vi "TCSLINK_global.vi"() -> ()   [LabVIEW 2015]
panel:
  out "Comp Mirror":bool
  in  "Dome":bool caption="Fe"
  out "Dome Percent":i8
  out "Quartz Percent":i8
  in  "Bulb":bool
  in  "Fe":bool
  in  "Quartz":bool
  in  "Ar":bool
  in  "Ne":bool
  in  "Cu":bool
  in  "Hg(Ar)":bool
  in  "Postion ADC":string
  in  "ObsDEC":string
  in  "ObsRA":string
  in  "Position Angle":dbl
  in  "Seeing":dbl
  in  "Humidity":dbl
  in  "Pressure":dbl
  in  "Wind Speed":dbl
  in  "Wind Direction":dbl
  in  "Outside Temp":dbl
  in  "Airmass":dbl
  in  "Focus":dbl
  in  "Rotator Location":string
  in  "Dome Shutter":string
  in  "Dome Az":dbl
  in  "Hour Angle":string
  in  "Sidereal Time":string
  in  "DEC":string
  in  "RA":string
  in  "Mount El":dbl
  in  "Mount Az":dbl
  in  "UT Time":string
  in  "Date":string
  in  "Rotator Angle":dbl
  out "TCSLink Online":bool
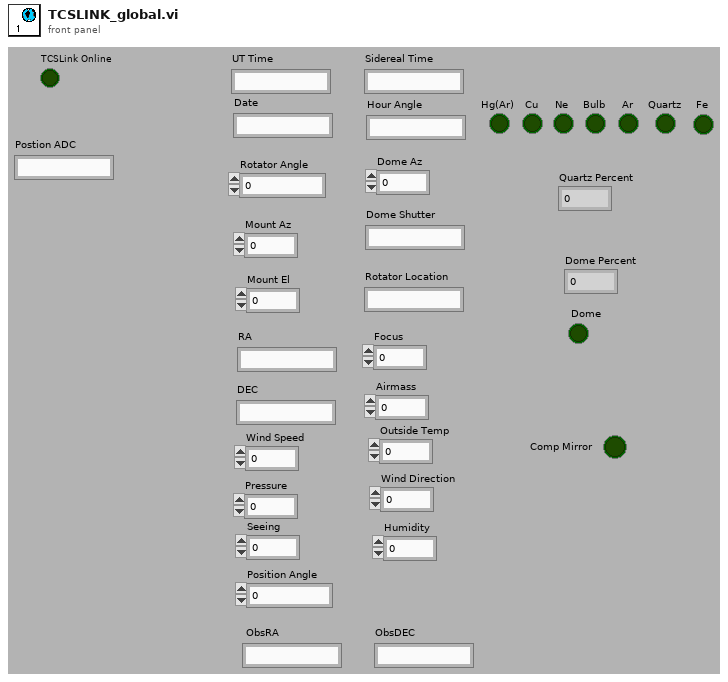
[diagram p1: front panel]
diagram:
